vi "Write Meta Data.vi"(7 "Unique ID":string, 8 "error in (no error)":errorcluster, 10 "Meta Data":string, 11 "Linked List in":refnum<class "Linked List.lvclass">) -> (0 "error out":errorcluster, 1 "Found?":bool, 3 "Linked List out":refnum<class "Linked List.lvclass">)   [LabVIEW 2020, in "Linked Lists.lvlib" / "Linked List.lvclass"]
uses:
  <vilib>/gpm_packages/@cs/linked-list/Source/Linked List/Linked List/Linked List.lvclass
  <vilib>/gpm_packages/@cs/linked-list/Source/Linked List/Linked List Definition/Linked List Definition.lvclass
  <vilib>/gpm_packages/@cs/linked-list/Source/Linked List/Linked List/Linked List.lvclass/Linked List.ctl
  <vilib>/gpm_packages/@cs/lookup-table/Source/LookupTable/LookupTable.lvclass/LookupTable.ctl
  e2f31741-640d-4f17-9c2b-5a311ae6dc2c.vi
  cce9c6bc-5a3f-403d-abaa-cce0601000c4.vi
  <vilib>/gpm_packages/@cs/lookup-table/Source/LookupTable/Read Table Reference.vi
  e2f31741-640d-4f17-9c2b-5a311ae6dc2c.vi/8e4ab30a-8150-4492-b9ab-9b4cb7717dec.vi
  cce9c6bc-5a3f-403d-abaa-cce0601000c4.vi/2e39944d-278f-4630-b5ee-6c48acbb6cc8.vi
  <vilib>/gpm_packages/@cs/lookup-table/Source/LookupTable/LookupTable.lvclass
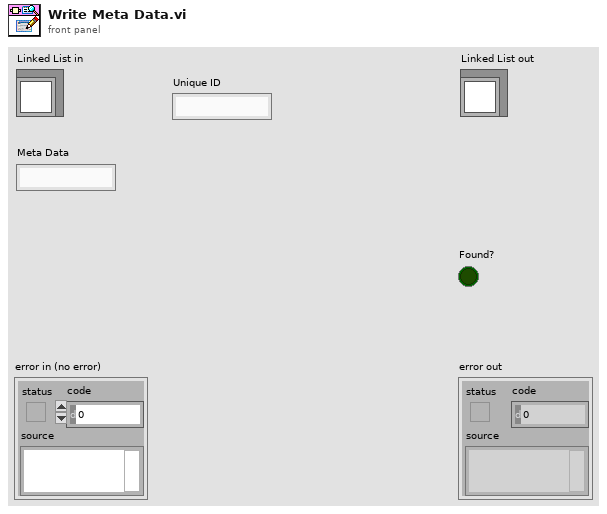
[diagram p1: front panel]
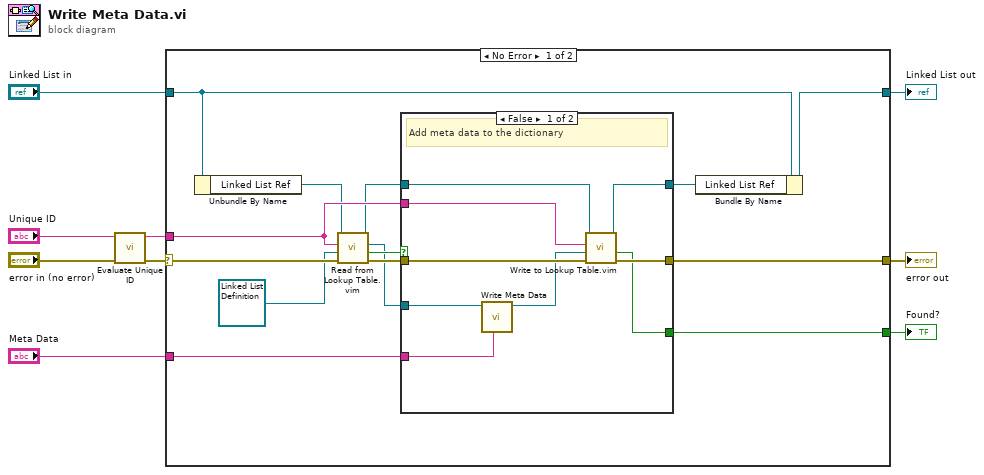
[diagram p0: block diagram]
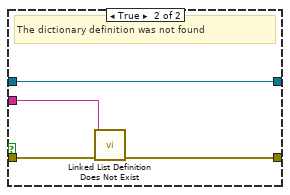
[diagram p2: hidden frame]
diagram:
  n1 = call <vilib>:"Evaluate Unique ID.vi"("error in (no error)"="error in (no error)", "Unique ID"="Unique ID") -> ("error out"=w8:errorcluster, "Unique ID Out"=w5:string)  [unwired: 8 in]
  n2 = case shown="No Error" w8 {
    selector: w8 -> [w23 w38]
    tunnel: [w19 w38] -> w7
    tunnel: w5 -> [w16 _]
    tunnel: [w11 w37] -> w4
    tunnel: "Linked List in" -> [w12 w37]
    tunnel: "Meta Data" -> [w17 _]
    tunnel: [w10 _] -> w1
    frame No Error {
      n3 = Unbundle By Name(w12) -> ("Linked List Ref"=w15:refnum<data-value>)
      n4 = call "Read from Lookup Table.vim"("error in (no error)"=w23, "Type"=refnum<class "Linked List Definition.lvclass"> refnum ("Linked List.lvlib:Linked List Definition.lvclass"), "Item Name"=w16, "LookupTable Reference"=w15) -> ("error out"=w20:errorcluster, "Not Found?"=w21:bool, "Value"=w18:refnum<class "Linked List Definition.lvclass">, "LookupTable Reference Out"=w14:refnum<data-value>)  [unwired: 4 in]
      n5 = case shown="False" w21 {
        tunnel: [w31 w35] -> w19
        tunnel: w20 -> [w32 w36]
        tunnel: w18 -> [w28 _]
        tunnel: w17 -> [w27 _]
        tunnel: w16 -> [w25 w34]
        tunnel: w14 -> [w30 w33]
        tunnel: [w29 w33] -> w13
        tunnel: [w24 _] -> w10
        frame False {
          # "Add meta data to the dictionary"
          n6 = call <vilib>:"Write Meta Data.vi"("Meta Data"=w27, "Linked List Definition in"=w28) -> ("Linked List Definition out"=w26:refnum<class "Linked List Definition.lvclass">)  [unwired: 9 in]
          n7 = call "Write to Lookup Table.vim"("error in (no error)"=w32, "Item"=w26, "Item Name"=w25, "LookupTable Reference"=w30) -> ("error out"=w31:errorcluster, "Replaced?"=w24:bool, "LookupTable Reference Out"=w29:refnum<data-value>)  [unwired: 5 in]
        }
        frame True {
          # "The dictionary definition was not found"
          n8 = call <vilib>:"Linked List Definition Does Not Exist.vi"("Error In"=w36, "Unique ID"=w34) -> ("Error Out"=w35:errorcluster)  [unwired: 9 in]
        }
      }
      n9 = Bundle By Name(cluster=w12, "Linked List Ref"=w13) -> (w11:refnum<class "Linked List.lvclass">)
    }
    frame Error {
    }
  }
  "error out" <- w7
  "Linked List out" <- w4
  "Found?" <- w1
